vi "Callback.vi"(7 "Owner":refnum<class>, 11 "Numeric":dbl) -> ()   [LabVIEW 2012, in "Callback Consumer.lvclass"]
uses:
  Callback Consumer.lvclass
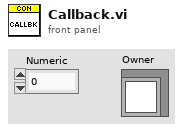
[diagram p1: front panel]
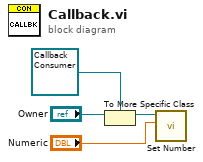
[diagram p0: block diagram]
diagram:
  n1 = To More Specific Class(target class=refnum<class "Callback Consumer.lvclass"> refnum ("Callback Consumer.lvclass"), reference="Owner") -> (specific class reference=w2:refnum<class "Callback Consumer.lvclass">)  [unwired: 1 in, 1 out]
  n2 = call "Set Number.vi"("Numeric"="Numeric", "Callback Consumer in"=w2) -> ()  [unwired: 8 in, 2 out]
